vi "Intensity Graph to Igor Graph.vi"(8 "error in (no error)":errorcluster, 9 "Filename":string="testname", 10 "Path":path=path "C:/temp", 11 "Intensity Graph Reference":refnum<vi>) -> (0 "error out":errorcluster, 2 "file":path)   [LabVIEW 2016, in "LV to ITX.lvclass"]
uses:
  LV to ITX.lvclass
  <userlib>/LevyLab/Graph Utilities/graph_utilities.lvclass/graph_utilities.ctl
  <userlib>/LevyLab/Graph Utilities/graph_utilities.lvclass
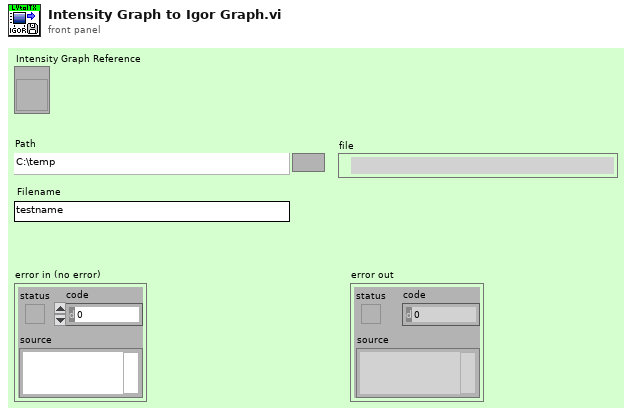
[diagram p1: front panel]
types:
  T1 = cluster{"Value":dbl[][], "X Scale":dbl[], "Y Scale":dbl[]}
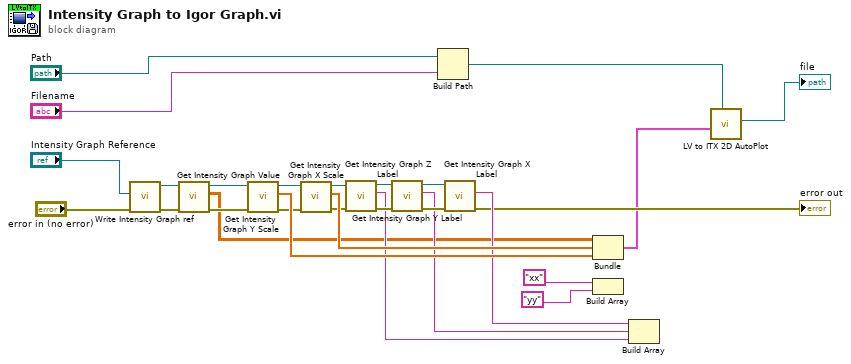
[diagram p0: block diagram]
diagram:
  n1 = call <userlib>:"Write Intensity Graph ref.vi"("error in (no error)"="error in (no error)", "Intensity Graph"="Intensity Graph Reference") -> ("error out"=w23:errorcluster, "graph_utilities out"=w24:refnum<class "graph_utilities.lvclass">)  [unwired: 8 in]
  n2 = call <userlib>:"Get Intensity Graph Value.vi"("error in (no error)"=w23, "graph_utilities in"=w24) -> ("error out"=w20:errorcluster, "Value"=w2:dbl[][], "graph_utilities out"=w21:refnum<class "graph_utilities.lvclass">)  [unwired: 7 in]
  n3 = call <userlib>:"Get Intensity Graph Y Scale.vi"("error in (no error)"=w20, "graph_utilities in"=w21) -> ("error out"=w17:errorcluster, "Y Scale"=w19:dbl[], "graph_utilities out"=w18:refnum<class "graph_utilities.lvclass">)  [unwired: 6 in, 1 out]
  n4 = call <userlib>:"Get Intensity Graph X Scale.vi"("error in (no error)"=w17, "graph_utilities in"=w18) -> ("error out"=w12:errorcluster, "X Scale"=w22:dbl[], "graph_utilities out"=w11:refnum<class "graph_utilities.lvclass">)  [unwired: 6 in, 1 out]
  n5 = call <userlib>:"Get Intensity Graph Z Label.vi"("error in (no error)"=w12, "graph_utilities in"=w11) -> ("error out"=w14:errorcluster, "Z Label"=w8:string, "graph_utilities out"=w13:refnum<class "graph_utilities.lvclass">)  [unwired: 7 in]
  n6 = call <userlib>:"Get Intensity Graph Y Label.vi"("error in (no error)"=w14, "graph_utilities in"=w13) -> ("error out"=w16:errorcluster, "Y Label"=w9:string, "graph_utilities out"=w15:refnum<class "graph_utilities.lvclass">)  [unwired: 7 in]
  n7 = Build Path(base path="Path", name or relative path="Filename") -> (appended path=w3:path)
  n8 = call <userlib>:"Get Intensity Graph X Label.vi"("error in (no error)"=w16, "graph_utilities in"=w15) -> ("error out"=→"error out":errorcluster, "X Label"=w10:string)  [unwired: 7 in, 1 out]
  n9 = Bundle("Value"=w2, "X Scale"=w22, "Y Scale"=w19) -> (w1:T1)  [unwired: 1 in]
  n10 = Build Array("xx" ("X Scale.Name Label.Text"), "yy" ("X Scale.Name Label.Text")) -> ()  [unwired: 1 out]
  n11 = Build Array(w10, w9, w8) -> ()  [unwired: 1 out]
  n12 = call "LV to ITX 2D AutoPlot.vi"("path"=w3, "2D, X, Y (Cluster)"=w1) -> ("file"=→"file":path)  [unwired: 7 in, 2 out]
